vi "Add New Line.vi"(8 "error in":errorcluster, 10 "Path":path, 11 "objects":T1) -> (0 "error out":errorcluster, 1 "success":bool, 2 "Line Index":i32)   [LabVIEW 2015, in "Sequencer Module editor node.lvclass"]
doc: "This VI is called to add new elements to the configuration. \nIt creates a new default line and the opens the dialog to edit its properties. \nFinally it adds it to the configuration."
uses:
  Sequencer Module editor node.lvclass
  <vilib>/NI/DCAF/Tag Editor Core/Table API/Table Manager/object ref.ctl
  <vilib>/NI/DCAF/Tag Editor Core/Configuration Editor/Classes/Engine Parent/Engine Parent Editor Node.lvclass
  <vilib>/NI/DCAF/Tag Editor Core/Configuration Editor/Classes/Module editor node/module editor node.lvclass
  Mappings.ctl
  module/configuration/Line.ctl
  classes/Sequence/Config/Sequence Config.lvclass
  Map.ctl
  <vilib>/NI/Tag Bus Module Framework/channel/TBM channel.lvclass
  <vilib>/Utility/file.llb/Read Delimited Spreadsheet (string).vi
  module/configuration/Sequencer Module configuration.lvclass
  <vilib>/NI/DCAF/Tag Editor Core/Table API/Table Manager/Table Manager.lvclass
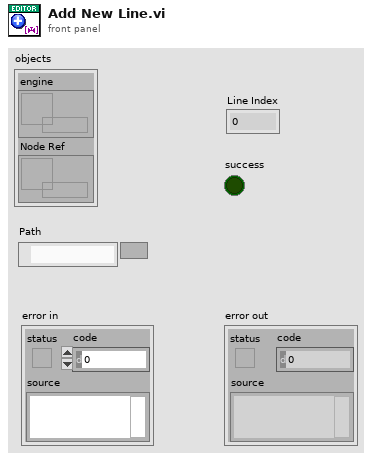
[diagram p1: front panel]
types:
  T1 = typedef "Table Manager.lvlib/Table Manager.lvclass/object ref.ctl" = cluster{"engine":refnum<data-value>, "Node Ref":refnum<data-value>}
  T2 = typedef "Sequencer Module editor node.lvclass/Mappings.ctl" = cluster{"Line":T3, "Maps":T4[]}
  T3 = typedef "Sequencer Module configuration.lvclass/Line.ctl" = cluster{"Sequence":refnum<class "Sequence Config.lvclass">}
  T4 = typedef "Sequencer Module editor node.lvclass/Map.ctl" = cluster{"channel":refnum<class "TBM channel.lvclass">, "tag name":string}
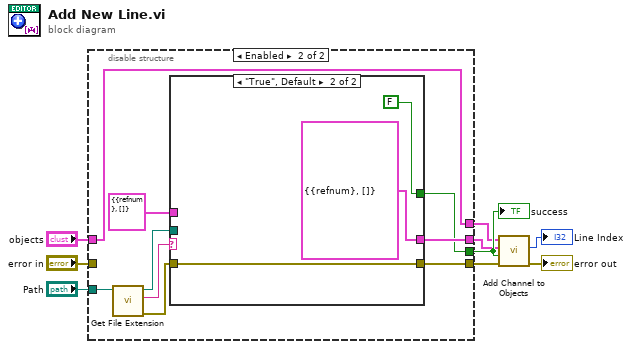
[diagram p0: block diagram]
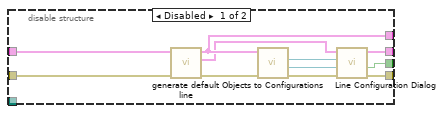
[diagram p2: hidden frame]
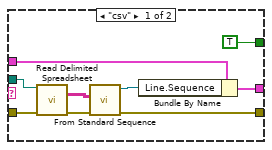
[diagram p3: hidden frame]
diagram:
  n1 = disable-structure shown="Enabled" {
    disable-tunnel: "objects" -> [w20 w29]
    disable-tunnel: "error in" -> [w19 _]
    disable-tunnel: [w18 w22] -> w7
    disable-tunnel: [w17 w21] -> w5
    disable-tunnel: [w16 w29] -> w4
    disable-tunnel: [w14 w24] -> w3
    disable-tunnel: "Path" -> [_ w28]
    frame Disabled {
      n2 = call "generate default line.vi"("error in"=w19, "objects in"=w20) -> ("error out"=w12:errorcluster, "Line"=w13:T3, "objects out"=w16:T1)  [unwired: 7 in]
      n3 = call "Objects to Configurations.vi"("error in (no error)"=w12, "Objects in"=w16) -> ("error out"=w15:errorcluster, "engine configuration out"=w10:refnum<class "engine configuration.lvclass">, "tag bus configurable plugin module configuration"=w11:refnum<class "Sequencer Module configuration.lvclass">)  [unwired: 7 in]
      n4 = call "Line Configuration Dialog.vi"("error in"=w15, "engine configuration in"=w10, "tag bus configurable plugin module configuration"=w11, "Line"=w13) -> ("error out"=w18:errorcluster, "success"=w17:bool, "Mappings out"=w14:T2)  [unwired: 4 in, 1 out]
    }
    frame Enabled {
      n5 = call <vilib>:"Get File Extension.vi"("file"=w28) -> ("error out"=w23:errorcluster, "lowercase file extension"=w27:string, "dup file"=w26:path)  [unwired: 6 in, 2 out]
      n6 = case shown="\"True\", Default" w27 {
        tunnel: w26 -> [w38 _]
        tunnel: T2 {"Line"={"Sequence"=refnum}, "Maps"=[]} ("Line Item in") -> [w36 _]
        tunnel: [w34 T2 {"Line"={"Sequence"=refnum}, "Maps"=[]} ("Line Item in")] -> w24
        tunnel: w23 -> [w33 w40]
        tunnel: [w31 w40] -> w22
        tunnel: [TRUE ("success") FALSE ("success")] -> w21
        frame "csv" {
          n7 = call-poly <vilib>:"Read Delimited Spreadsheet.vi"("file path (dialog if empty)"=w38, "error in (no error)"=w33) -> ("all rows"=w37:string[][], "error out"=w32:errorcluster)  [unwired: 8 in, 4 out]
          n8 = call "From Standard Sequence.vi"("error in (no error)"=w32, "Standard Sequence"=w37) -> ("error out"=w31:errorcluster, "Sequence Config.lvclass"=w35:refnum<class "Sequence Config.lvclass">)  [unwired: 8 in]
          n9 = Bundle By Name(cluster=w36, "Line.Sequence"=w35) -> (w34:T2)
        }
        frame "True", Default {
        }
      }
    }
  }
  "success" <- w5
  n10 = call "Add Channel to Objects.vi"("error in"=w7, "Add? (T)"=w5, "Line Item in"=w3, "Objects in"=w4) -> ("error out"=→"error out":errorcluster, "Line Index"=→"Line Index":i32)  [unwired: 6 in]
